vi "SVA 4MV6 T023 CCE.vi"() -> ()   [LabVIEW 2020]
doc: "Ceballos Conde Emanuel 4MV6 Sistemas de visión artificial 2022/1\nEste vi contiene un SISTEMA MIMO AUTONOMO basado en arreglos como se planteo en clase"
panel:
  out "output values":dbl[](array[numeric])
  out "distancia":dbl(slide) scale=0.0..100.0
  out "angulo":dbl(knob) scale=-25.0..25.0
  in  "Reset":bool
  out "Motor Izquierda":dbl(slide) scale=-100.0..100.0
  out "Motor Derecha":dbl(slide) scale=-100.0..100.0
  out "Plano de trabajo":picture
  in  "stop":bool
  # "Ceballos Conde Emanuel\n4MV6\nSistemas de visión artificial\n2022/1"
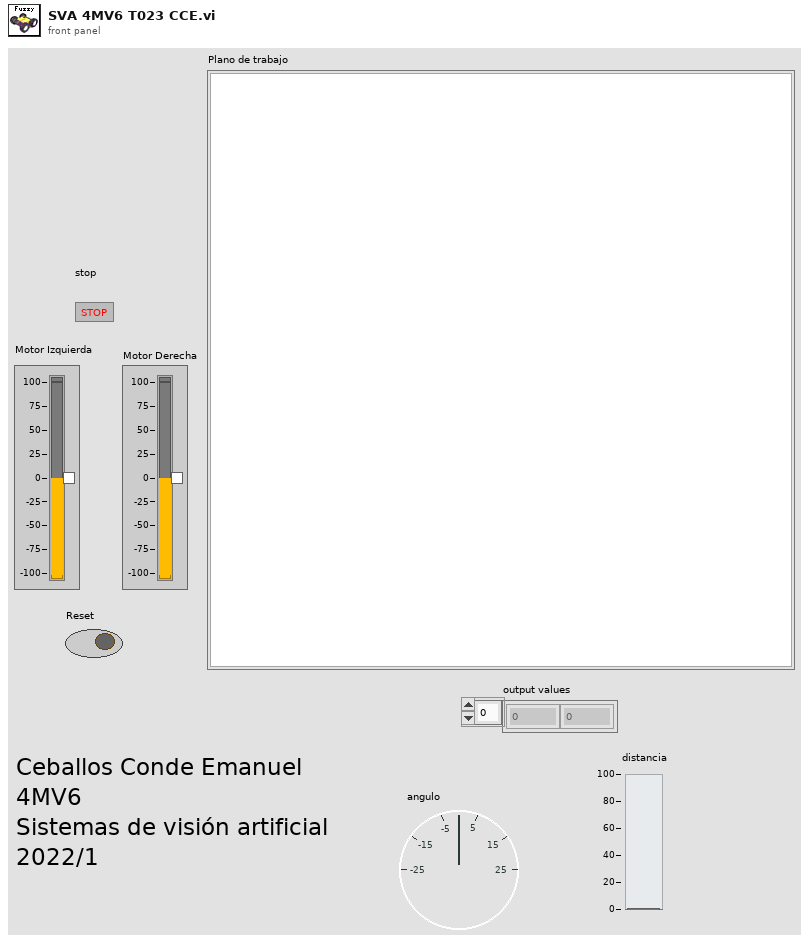
[diagram p1: front panel]
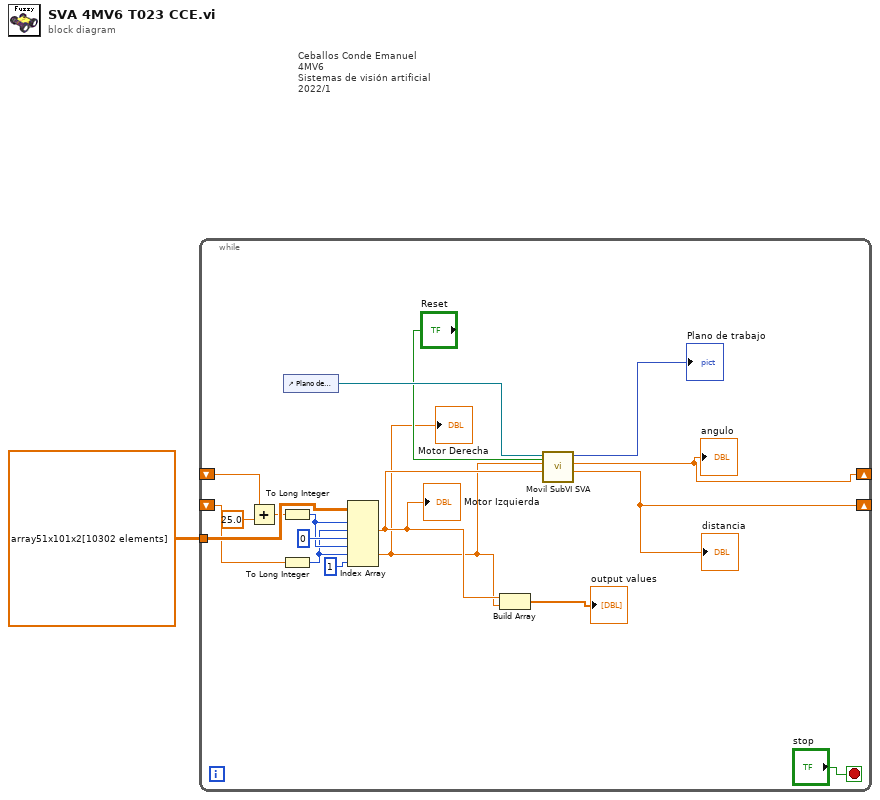
[diagram p0: block diagram]
diagram:
  # "Ceballos Conde Emanuel\n4MV6\nSistemas de visión artificial\n2022/1"
  n1 = while {
    tunnel: dbl[][][] array51x101x2[10302 elements] ("output values 2") -> [w14]
    shift-right: [w10] -> _
    shift-left: _ -> [w9]
    shift-right: [w2] -> _
    shift-left: _ -> [w8]
    stop <- "stop" stop-if-true
    n2 = Add(x=w9, y=25.0) -> (x+y=w11:dbl)
    n3 = To Long Integer(number=w11) -> (32bit integer=w7:i32)
    n4 = To Long Integer(number=w8) -> (32bit integer=w6:i32)
    n5 = control-ref of="Plano de trabajo"() -> (w17:refnum<vi>)
    n6 = Index Array(array=w14, index (dim 0) #1=w7, index (dim 1) #1=w6, index (dim 2) #1=0 ("disabled index (col)"), index (dim 0) #2=w7, index (dim 1) #2=w6, index (dim 2) #2=1 ("disabled index (col)")) -> (element #1=w5:dbl, element #2=w4:dbl)
    "Motor Derecha" <- w4
    "Motor Izquierda" <- w5
    n7 = Build Array(w5, w4) -> (→"output values":dbl[])
    n8 = call "Movil SubVI SVA.vi"("Reset"="Reset", "Motor Izquierda"=w5, "Motor Derecha"=w4, "Ref Plano"=w17) -> ("Distancia"=w2:dbl, "Angulo"=w10:dbl, "Plano de trabajo"=→"Plano de trabajo":picture)  [unwired: 3 in, 2 out]
    "distancia" <- w2
    "angulo" <- w10
  }
